vi "left_side_centralize.vi"(0 "samples":i32, 1 "step(mm)":i32, 2 "inner_b_ir":dbl, 3 "inner_f_ir":dbl) -> ()   [LabVIEW 2017]
uses:
  <vilib>/myRIO/Instrument Drivers/Onboard IO/AI/typedefs/AI Reference.ctl
  <vilib>/myRIO/Common/Instrument Driver Framework/Utilities/typedefs/myRIO Generic Hardware Reference.ctl
  <vilib>/myRIO/Common/Instrument Driver Framework/Utilities/typedefs/Hardware Version Enum.ctl
  <vilib>/myRIO/Common/Instrument Driver Framework/Utilities/typedefs/myRIO v1.0 Reference.ctl
  <vilib>/myRIO/Common/Instrument Driver Framework/Utilities/typedefs/Generic FPGA Reference.ctl
  <vilib>/myRIO/Common/Instrument Driver Framework/myRIO v1.0/AI/typedefs/AI Channels List.ctl
  <vilib>/myRIO/Common/Instrument Driver Framework/myRIO v1.0/AI/typedefs/AI Channels Enum.ctl
  <vilib>/myRIO/Common/Instrument Driver Framework/Utilities/typedefs/Analog Scaling Constants List.ctl
  <vilib>/myRIO/Common/Instrument Driver Framework/Utilities/typedefs/Analog Scaling Constants.ctl
  <vilib>/userdefined/High Color/nirio_resource_hc.ctl
  <vilib>/myRIO/Common/Instrument Driver Framework/Utilities/vis/Is FPGA Ref Available.vi
  <vilib>/myRIO/Common/Instrument Driver Framework/myRIO v1.0/AI/vis/myRIO v1.1 Open AI.vi
  <vilib>/myRIO/Instrument Drivers/Onboard IO/AI/vis/Read.vi
  <vilib>/Analysis/baseanly.llb/Mean (DBL).vi
  <vilib>/myRIO/Common/Instrument Driver Framework/Utilities/vis/Validate Channels.vi
  <vilib>/myRIO/Common/Instrument Driver Framework/myRIO v1.0/AI/vis/myRIO v1.0 Reserve AI.vi
  <vilib>/myRIO/Common/Instrument Driver Framework/myRIO v1.0/AI/vis/myRIO v1.0 Build MUX Configuration AI.vi
  <vilib>/myRIO/Common/Instrument Driver Framework/myRIO v1.0/Resource Manager/vis/myRIO v1.0 Reserve Channel List.vi
  <vilib>/myRIO/Common/Instrument Driver Framework/myRIO v1.0/Resource Manager/vis/myRIO v1.0 Reserve Channel.vi
  <vilib>/myRIO/Common/Instrument Driver Framework/myRIO v1.0/Resource Manager/vis/myRIO v1.0 Unreserve Channel.vi
  <vilib>/myRIO/Common/Instrument Driver Framework/myRIO v1.0/Resource Manager/vis/myRIO v1.0 Build Mutex Name.vi
  <vilib>/Utility/VariantDataType/GetNumericInfo.vi
  <vilib>/Utility/error.llb/Error Cluster From Error Code.vi
  <vilib>/myRIO/Common/Instrument Driver Framework/myRIO v1.0/myRIO v1.1 Open.vi
  <vilib>/myRIO/Common/Instrument Driver Framework/myRIO v1.0/AI/vis/myRIO v1.0 Get Scaling Constants AI.vi
  <vilib>/myRIO/Common/Instrument Driver Framework/Utilities/vis/IO Manager.vi
  <vilib>/myRIO/Common/Instrument Driver Framework/Utilities/vis/Configuration Manager.vi
  <vilib>/myRIO/Common/Instrument Driver Framework/myRIO v1.0/myRIO v1.0 Close.vi
  <vilib>/myRIO/Common/Instrument Driver Framework/myRIO v1.0/AI/vis/myRIO v1.0 Read AI.vi
  GlobalVar.vi
  <vilib>/myRIO/Express VI/Onboard IO/AI/AI Express VI.xnode
  <vilib>/myRIO/Instrument Drivers/Onboard IO/AI/vis/myRIO AI Open.xnode
  <vilib>/Analysis/NI_AALBase.lvlib
  <vilib>/myRIO/Instrument Drivers/Onboard IO/AI/AI.lvlib
panel:
  out "pre_r":i32
  out "pre_l":i32
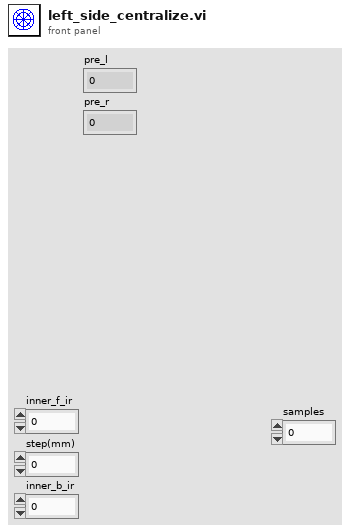
[diagram p1: front panel]
types:
  T1 = typedef "AI.lvlib/AI Reference.ctl" = cluster{"myRIO Reference":T2, "AI Channels List":T6, "AI Scaling Constants List":T8}
  T2 = typedef "myRIO Generic Hardware Reference.ctl" = cluster{"myRIO Model":T3, "myRIO Hardware Reference":T4}
  T3 = typedef "Hardware Version Enum.ctl" = enum16{"Unknown", "myRIO-1900", "myRIO-1950", "roboRIO", "NI ELVIS RIO CM"}
  T4 = typedef "myRIO v1.0 Reference.ctl" = cluster{"Generic FPGA Reference":T5, "Allow multiple opens":bool}
  T5 = typedef "Generic FPGA Reference.ctl" = refnum<k20>
  T6 = typedef "AI Channels List.ctl" = T7[]
  T7 = typedef "AI Channels Enum.ctl" = enum16{"Not Connected", "AudioIn/Left", "AudioIn/Right", "C/AI0", "C/AI1", "A/AI0", "A/AI1", "A/AI2", "A/AI3", "B/AI0", "B/AI1", "B/AI2", "B/AI3", "AI/AI0", "AI/AI1", "AI/AI2", "AI/AI3"}
  T8 = typedef "Analog Scaling Constants List.ctl" = T9[]
  T9 = typedef "Analog Scaling Constants.ctl" = cluster{"LSB Weight (Volts)":dbl, "Offset (Volts)":dbl, "Signed?":bool}
  T10 = typedef "nirio_resource_hc.ctl" = tag
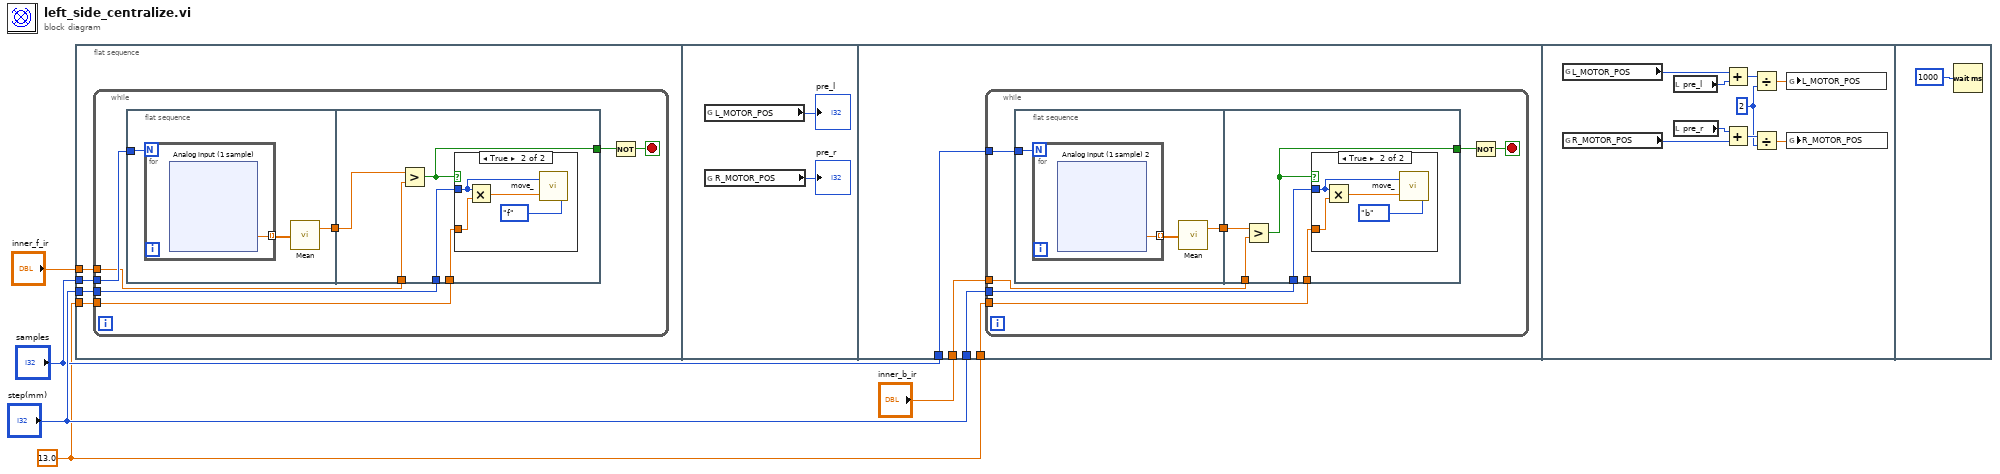
[diagram p0: block diagram]
diagram:
  w1 = 13.0 ("y")
  n1 = flat-sequence {
    tunnel: "samples" -> [w9]
    tunnel: "inner_f_ir" -> [w8]
    tunnel: "step(mm)" -> [w7]
    tunnel: w1 -> [w6]
    tunnel: "step(mm)" -> [w72]
    tunnel: "inner_b_ir" -> [w71]
    tunnel: "samples" -> [w70]
    tunnel: w1 -> [w69]
    frame #0 {
      n2 = while {
        tunnel: w9 -> [w16]
        tunnel: w8 -> [w14]
        tunnel: w7 -> [w13]
        tunnel: w6 -> [w10]
        stop <- w12 stop-if-true
        n3 = flat-sequence {
          tunnel: w16 -> [w18]
          tunnel: [w17] -> w15
          tunnel: w15 -> [w62]
          tunnel: w14 -> [w61]
          tunnel: w13 -> [w60]
          tunnel: [w59] -> w11
          tunnel: w10 -> [w58]
          frame #0 {
            n4 = for {
              N: w18 -> [_]
              tunnel: [w20] -> w19 mode=indexing
              n5 = xnode "Analog input (1 sample)"() -> ("lf (B/AI2 (Pin 7))"=w20:dbl)  [unwired: 1 in, 1 out]
            }
            n6 = call-poly <vilib>:"Mean.vi"("X"=w19) -> ("mean"=w17:dbl)  [unwired: 1 out]
          }
          frame #1 {
            n7 = Greater?(x=w62, y=w61) -> (0:w59:bool)
            n8 = case shown="True" w59 {
              tunnel: w60 -> [_ w64]
              tunnel: w58 -> [_ w63]
              frame False {
              }
              frame True {
                n9 = Multiply(x=w64, y=w63) -> (x*y=w65:dbl)
                n10 = call "move_.vi"("Enum"=enum16{"hold", "f", "b"}."f", "delay"=w65, "D"=w64) -> ()  [unwired: 1 in]
              }
            }
          }
        }
        n11 = Not(x=w11) -> (.not. x?=w12:bool)
      }
    }
    frame #1 {
      n12 = global read "GlobalVar.vi" "L_MOTOR_POS"() -> (→"pre_l":i32)
      n13 = global read "GlobalVar.vi" "R_MOTOR_POS"() -> (→"pre_r":i32)
    }
    frame #2 {
      n14 = while {
        tunnel: w72 -> [w78]
        tunnel: w71 -> [w75]
        tunnel: w70 -> [w74]
        tunnel: w69 -> [w73]
        stop <- w77 stop-if-true
        n15 = flat-sequence {
          tunnel: [w82] -> w79
          tunnel: w74 -> [w80]
          tunnel: w79 -> [w125]
          tunnel: w78 -> [w124]
          tunnel: [w123] -> w76
          tunnel: w75 -> [w122]
          tunnel: w73 -> [w121]
          frame #0 {
            n16 = for {
              N: w80 -> [_]
              tunnel: [w83] -> w81 mode=indexing
              n17 = xnode "Analog input (1 sample) 2"() -> ("lb (B/AI3 (Pin 9))"=w83:dbl)  [unwired: 1 in, 1 out]
            }
            n18 = call-poly <vilib>:"Mean.vi"("X"=w81) -> ("mean"=w82:dbl)  [unwired: 1 out]
          }
          frame #1 {
            n19 = Greater?(x=w125, y=w122) -> (0:w123:bool)
            n20 = case shown="True" w123 {
              tunnel: w124 -> [_ w127]
              tunnel: w121 -> [_ w126]
              frame False {
              }
              frame True {
                n21 = Multiply(x=w127, y=w126) -> (x*y=w128:dbl)
                n22 = call "move_.vi"("Enum"=enum16{"hold", "f", "b"}."b", "delay"=w128, "D"=w127) -> ()  [unwired: 1 in]
              }
            }
          }
        }
        n23 = Not(x=w76) -> (.not. x?=w77:bool)
      }
    }
    frame #3 {
      w132 = 2 ("y")
      n24 = global read "GlobalVar.vi" "L_MOTOR_POS"() -> (w138:i32)
      n25 = global read "GlobalVar.vi" "R_MOTOR_POS"() -> (w137:i32)
      n26 = local read "pre_l"() -> (w136:i32)
      n27 = local read "pre_r"() -> (w135:i32)
      n28 = Add(x=w138, y=w136) -> (x+y=w134:i32)
      n29 = Add(x=w135, y=w137) -> (x+y=w133:i32)
      n30 = Divide(x=w134, y=w132) -> (x/y=w130:dbl)
      n31 = Divide(x=w133, y=w132) -> (x/y=w131:dbl)
      n32 = global write "GlobalVar.vi" "L_MOTOR_POS"(w130) -> ()
      n33 = global write "GlobalVar.vi" "R_MOTOR_POS"(w131) -> ()
    }
    frame #4 {
      n34 = Wait (ms)(milliseconds to wait=u32 1000) -> ()  [unwired: 1 out]
    }
  }
